vi "DisplaySequenceCallback.vi"(4 "output cluster":T1, 5 "Event Data":cluster{"file":refnum<k7>, "reason":i32}, 6 "Control Ref":refnum<k7>, 7 "Event Common Data":T2) -> ()   [LabVIEW 2010]
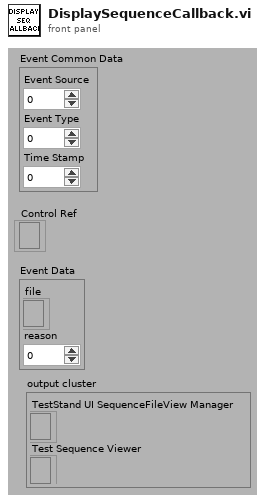
[diagram p1: front panel]
types:
  T1 = cluster{"TestStand UI SequenceFileView Manager":refnum<k7>, "Test Sequence Viewer":refnum<k7>}
  T2 = cluster{"Event Source":i32, "Event Type":u32, "Time Stamp":u32}
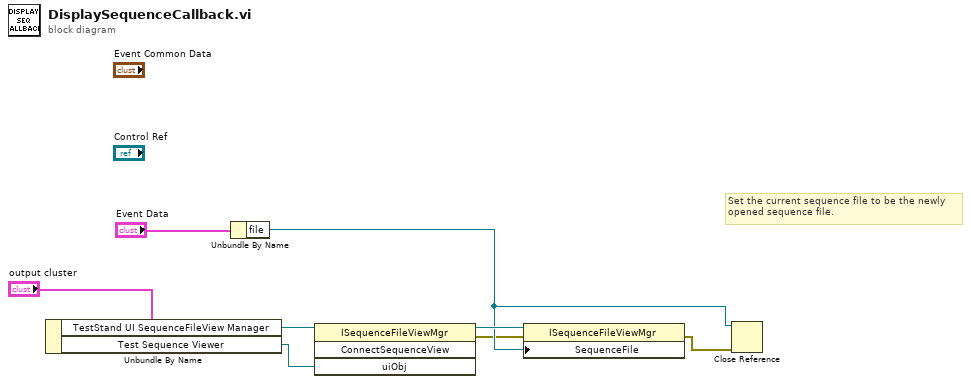
[diagram p0: block diagram]
diagram:
  # "Set the current sequence file to be the newly\nopened sequence file."
  n1 = Unbundle By Name("output cluster") -> ("TestStand UI SequenceFileView Manager"=w6:refnum<k7>, "Test Sequence Viewer"=w4:refnum<k7>)
  n2 = Unbundle By Name("Event Data") -> ("file"=w2:refnum<k7>)
  n3 = invoke class="ISequenceFileViewMgr" method="ConnectSequenceView"(reference=w6, "uiObj"=w4) -> (reference out=w5:refnum<k7>, error out=w1:errorcluster)  [unwired: 2 in, 2 out]
  n4 = property class="ISequenceFileViewMgr"(reference=w5, error in=w1, "SequenceFile"=w2) -> (error out=w3:errorcluster)  [unwired: 1 out]
  n5 = Close Reference(reference=w2, error in (no error)=w3) -> ()  [unwired: 1 out]
